vi "convertPhysicalChannels.vi"(8 "error in (no error)":errorcluster, 10 "Physical Channels":string, 11 "DIO64Output in":refnum<class "DIO64Output.lvclass">) -> (0 "error out":errorcluster, 1 "mask":u16[](array[numeric])=[1] format="%.0x", 2 "#ports":u8=1 min=1 max=8, 3 "DIO64Output out":refnum<class "DIO64Output.lvclass">)   [LabVIEW 2009, in "Hardware.lvlib" / "Channels.lvlib" / "DIO64Output.lvclass"]
uses:
  DIO64Output.lvclass
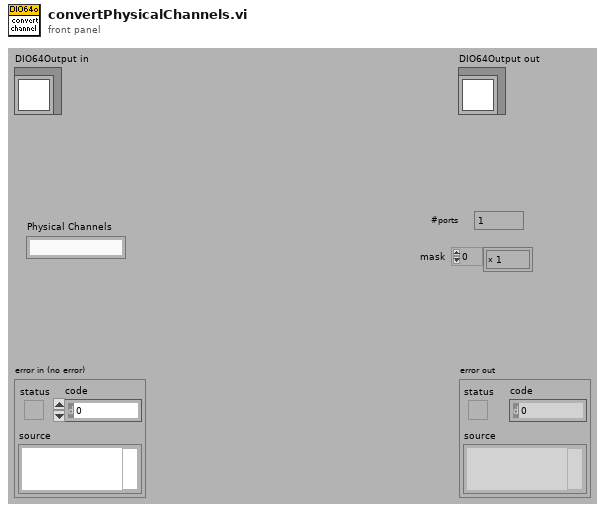
[diagram p1: front panel]
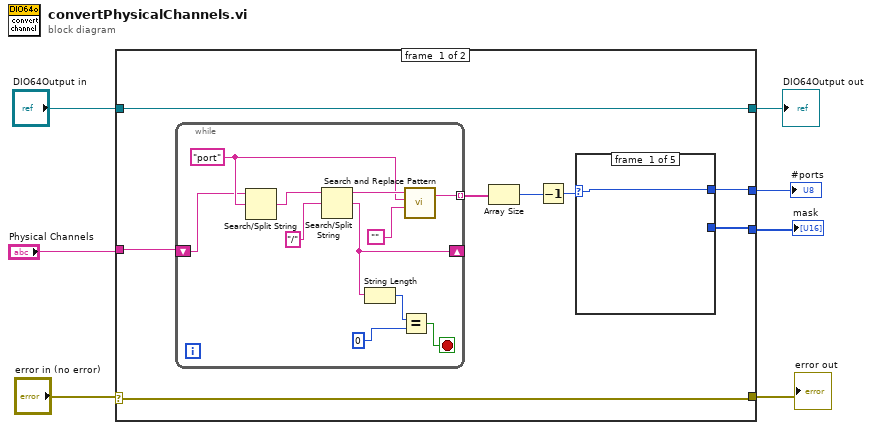
[diagram p0: block diagram]
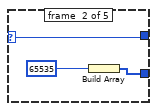
[diagram p2: hidden frame]
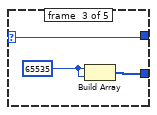
[diagram p3: hidden frame]
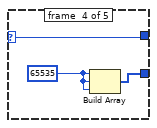
[diagram p4: hidden frame]
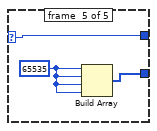
[diagram p5: hidden frame]
diagram:
  n1 = case shown="No Error" "error in (no error)" {
    selector: "error in (no error)" -> [w14 w41]
    tunnel: [w14 w41] -> w6
    tunnel: [w15 w40] -> w4
    tunnel: "DIO64Output in" -> [w15 w40]
    tunnel: "Physical Channels" -> [w12 _]
    tunnel: [w13 _] -> w2
    tunnel: [w8 _] -> w1
    frame #0 {
      n2 = while {
        tunnel: [w21] -> w10 mode=indexing
        shift-right: [w19] -> _
        shift-left: w12 -> [w20]
        stop <- w16 stop-if-true
        w23 = "port"
        n3 = Search/Split String(string=w20, search string/char (-)=w23) -> (match + rest of string=w26:string)  [unwired: 1 in, 2 out]
        n4 = Search/Split String(string=w26, search string/char (-)="/") -> (substring before match=w24:string, match + rest of string=w19:string)  [unwired: 1 in, 1 out]
        n5 = String Length(string=w19) -> (length=w18:i32)
        n6 = Equal?(x=w18, y=0) -> (x = y?=w16:bool)
        n7 = call <vilib>:"Search and Replace Pattern.vi"("string"=w24, "regular expression (\"\")"=w23, "replace string (\"\")"="") -> ("result string"=w21:string)  [unwired: 2 in, 1 out]
      }
      n8 = Array Size(array=w10) -> (size(s)=w11:i32)
      n9 = Decrement(x=w11) -> (x-1=w9:i32)
      n10 = case shown="1" w9 {
        selector: w9 -> [w27 w28 w31 w34 w37]
        tunnel: [_ w29 w32 w35 w38] -> w13
        tunnel: [w27 w28 w31 w34 w37] -> w8
        frame #0 {
        }
        frame #1 {
          n11 = Build Array(u16 65535) -> (w29:u16[])
        }
        frame #2 {
          w33 = u16 65535
          n12 = Build Array(w33, w33) -> (w32:u16[])
        }
        frame #3 {
          w36 = u16 65535
          n13 = Build Array(w36, w36, w36) -> (w35:u16[])
        }
        frame #4 {
          w39 = u16 65535
          n14 = Build Array(w39, w39, w39, w39) -> (w38:u16[])
        }
      }
    }
    frame #1 {
    }
  }
  "error out" <- w6
  "DIO64Output out" <- w4
  "#ports" <- w1
  "mask" <- w2
